vi "ForwardVision.vi"(11 "RobotDriveDevRef":T1={"DevStatus"={"status"=FALSE, "code"=0, "source"=""}, "Motors[]"=[], "Square Inputs"=FALSE, "Max Output"=1.0}) -> (3 "RobotDriveDevRef 2":T1={"DevStatus"={"status"=FALSE, "code"=0, "source"=""}, "Motors[]"=[], "Square Inputs"=FALSE, "Max Output"=1.0})   [LabVIEW 2016]
uses:
  <vilib>/Rock Robotics/WPI/RobotDrive/WPI_RobotDriveDevRef.ctl
  <vilib>/Rock Robotics/WPI/MotorControl/WPI_MotorControlDeviceRef.ctl
  <vilib>/Rock Robotics/WPI/MotorControl/WPI_MotorControlType.ctl
  <vilib>/Rock Robotics/SystemInterfaces/DIO/FPGA_DIOPWMChannel.ctl
  <vilib>/Rock Robotics/WPI/PWM/WPI_PWMDeadband.ctl
  Robot Global Data.vi
  <vilib>/Rock Robotics/WPI/RobotDrive/WPI_RobotDriveArcadeDrive_Standard(NoSaturation).vi
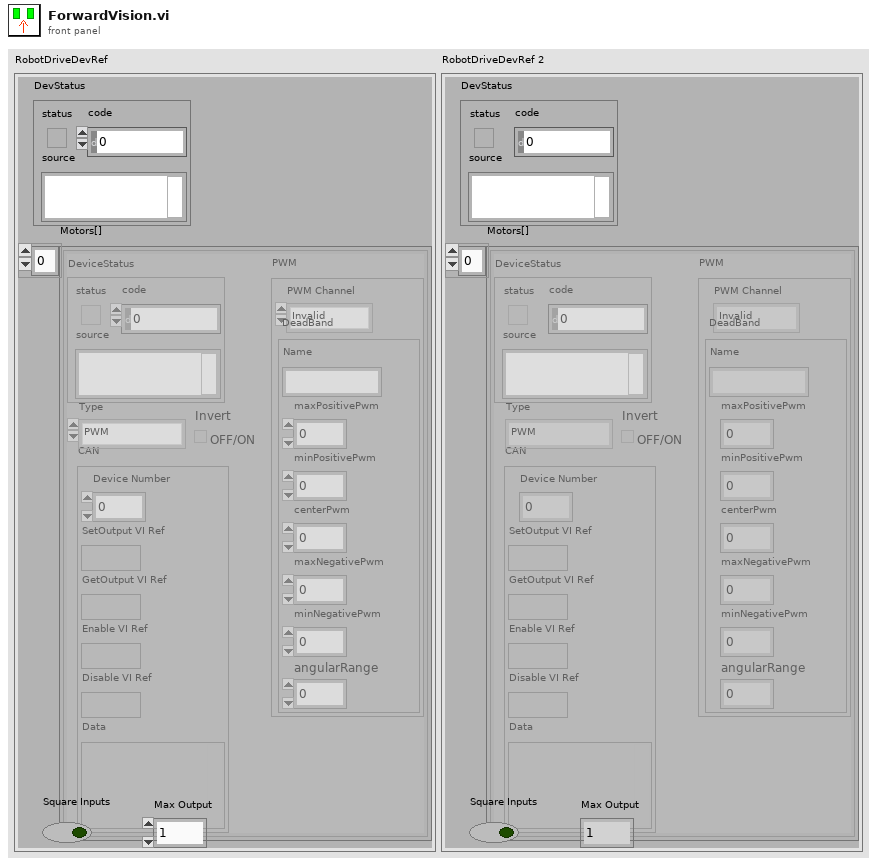
[diagram p1: front panel]
types:
  T1 = typedef "WPI_RobotDriveDevRef.ctl" = cluster{"DevStatus":errorcluster, "Motors[]":T2[], "Square Inputs":bool, "Max Output":dbl}
  T2 = typedef "WPI_MotorControlDeviceRef.ctl" = cluster{"DeviceStatus":errorcluster, "Type":T3, "PWM":cluster{"PWM Channel":T4, "DeadBand":T5}, "CAN":cluster{"Device Number":u8, "SetOutput VI Ref":variant, "GetOutput VI Ref":variant, "Enable VI Ref":variant, "Disable VI Ref":variant, "Data":variant}, "Invert":bool}
  T3 = typedef "WPI_MotorControlType.ctl" = enum16{"PWM", "CAN"}
  T4 = typedef "FPGA_DIOPWMChannel.ctl" = enum8{"PWM 0", "PWM 1", "PWM 2", "PWM 3", "PWM 4", "PWM 5", "PWM 6", "PWM 7", "PWM 8", "PWM 9", "PWM MXP 0", "PWM MXP 1", "PWM MXP 2", "PWM MXP 3", "PWM MXP 4", "PWM MXP 5", "PWM MXP 6", "PWM MXP 7", "PWM MXP 8", "PWM MXP 9", "Invalid"}
  T5 = typedef "WPI_PWMDeadband.ctl" = cluster{"Name":string, "maxPositivePwm":i32, "minPositivePwm":i32, "centerPwm":i32, "maxNegativePwm":i32, "minNegativePwm":i32, "angularRange":u16}
  T6 = cluster{"Lower X":dbl, "Lower Y":dbl, "Upper X":dbl, "Upper Y":dbl, "Lower Limit":dbl, "Upper Limit":dbl}
  T7 = cluster{"Target?":bool, "PegAngle":dbl, "Distance":dbl}
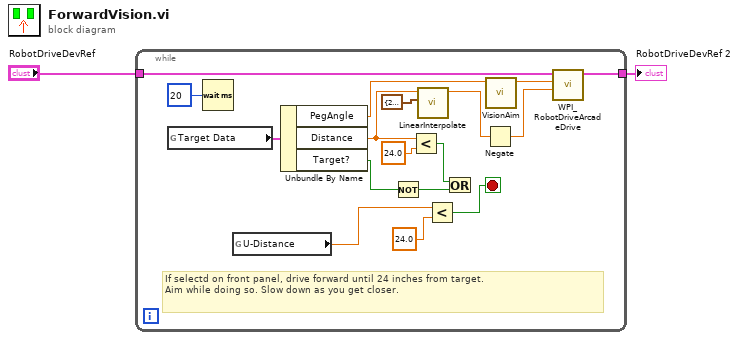
[diagram p0: block diagram]
diagram:
  n1 = while {
    tunnel: "RobotDriveDevRef" -> [w18]
    tunnel: [w17] -> w2
    stop <- w3 stop-if-true
    # "If selectd on front panel, drive forward until 24 inches from target.\nAim while doing so. Slow down as you get closer."
    n2 = global read "Robot Global Data.vi" "Target Data"() -> (w13:T7)
    n3 = Wait (ms)(milliseconds to wait=u32 20) -> ()  [unwired: 1 out]
    n4 = global read "Robot Global Data.vi" "U-Distance"() -> (w5:dbl)
    n5 = Unbundle By Name(w13) -> ("PegAngle"=w12:dbl, "Distance"=w7:dbl, "Target?"=w9:bool)
    n6 = Not(x=w9) -> (.not. x?=w10:bool)
    n7 = Less?(x=w7, y=24.0) -> (x < y?=w11:bool)
    n8 = call "LinearInterpolate.vi"("Config"=T6 {"Lower X"=24.0, "Lower Y"=0.48, "Upper X"=65.0, "Upper Y"=0.8, "Lower Limit"=0.45, "Upper Limit"=0.75}, "Value"=w7) -> ("Ouput"=w6:dbl)  [unwired: 9 in]
    n9 = Less?(x=w5, y=24.0) -> (x < y?=w3:bool)
    n10 = Or(x=w11, y=w10) -> ()  [unwired: 1 out]
    n11 = Negate(x=w6) -> (-x=w14:dbl)
    n12 = call "VisionAim.vi"("Angle"=w12) -> ("Turn Amount"=w19:dbl)  [unwired: 9 in, 1 out]
    n13 = call-poly <vilib>:"WPI_RobotDriveArcadeDrive.vi"("Y axis value"=w14, "X axis value"=w19, "RobotDriveDevRef"=w18) -> ("RobotDriveDevRef"=w17:T1)  [unwired: 6 in, 2 out]
  }
  "RobotDriveDevRef 2" <- w2
